vi "Read Output Values.vi"(0 "VISA resource name":refnum<visa-resource-name>, 1 "Unit Address (1)":u8=1 min=1 max=254, 11 "error in (no error)":errorcluster) -> (4 "VISA resource name out":refnum<visa-resource-name>, 10 "Manual Output Value":sgl, 15 "error out":errorcluster)   [LabVIEW 2010, in "Eurotherm 32xx Series.lvlib"]
doc: "This VI returns Output Values."
uses:
  <instrlib>/Eurotherm 32xx Series/Eurotherm 32xx Series.lvlib
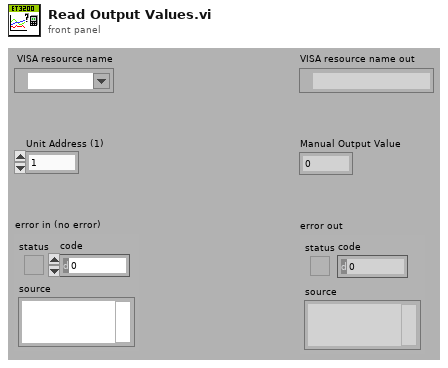
[diagram p1: front panel]
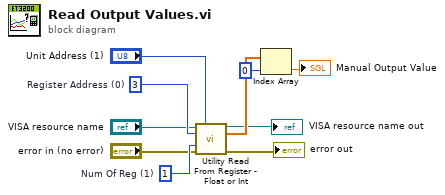
[diagram p0: block diagram]
diagram:
  w7 = u16 3  # Register Address (0)
  w8 = u16 1  # Num Of Reg (1)
  n1 = call <instrlib>:"Utility Read From Register - Float or Int.vi"("VISA resource name"="VISA resource name", "Unit Address (1)"="Unit Address (1)", "Register Address (0)"=w7, "Num Of Reg (1)"=w8, "error in (no error)"="error in (no error)") -> ("VISA resource name out"=→"VISA resource name out":refnum<visa-resource-name>, "Data"=w9:sgl[], "error out"=→"error out":errorcluster)  [unwired: 8 in]
  n2 = Index Array(array=w9, index=0) -> (element=→"Manual Output Value":sgl)
